vi "Initialize.vi"(8 "error in (no error)":errorcluster, 11 "Software Lock-in in":refnum<class "Software Lock-in.lvclass">) -> (0 "error out":errorcluster, 3 "Software Lock-in out":refnum<class "Software Lock-in.lvclass">)   [LabVIEW 2016, in "Software Lock-in.lvclass"]
uses:
  Software Lock-in.lvclass
  Software Lock-in.lvclass/Software Lock-in.ctl
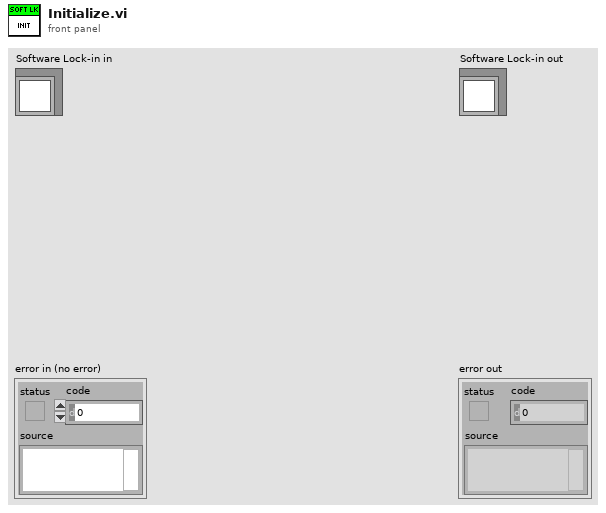
[diagram p1: front panel]
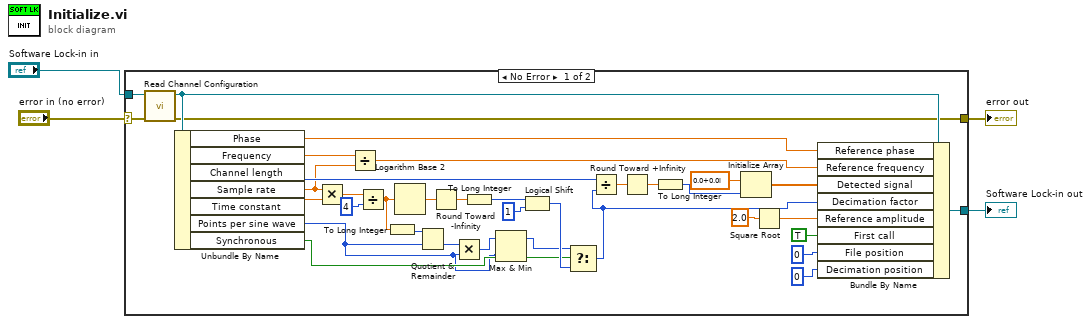
[diagram p0: block diagram]
diagram:
  n1 = case shown="No Error" "error in (no error)" {
    selector: "error in (no error)" -> [w36 w42]
    tunnel: [w25 w42] -> w3
    tunnel: [w39 w41] -> w1
    tunnel: "Software Lock-in in" -> [w40 w41]
    frame No Error {
      n2 = call-dynamic "Read Channel Configuration.vi"("error in (no error)"=w36, "Software Lock-in in"=w40) -> ("error out"=w25:errorcluster, "Software Lock-in out"=w35:refnum<class "Software Lock-in.lvclass">)  [unwired: 8 in]
      n3 = Unbundle By Name(w35) -> ("Phase"=w32:dbl, "Frequency"=w16:dbl, "Channel length"=w24:i64, "Sample rate"=w14:dbl, "Time constant"=w17:dbl, "Points per sine wave"=w7:i32, "Synchronous"=w9:bool)
      n4 = Multiply(x=w14, y=w17) -> (x*y=w31:dbl)
      n5 = Divide(x=w16, y=w14) -> (x/y=w15:dbl)
      n6 = Divide(x=w31, y=4) -> (x/y=w11:dbl)
      n7 = To Long Integer(number=w11) -> (32bit integer=w12:i32)
      n8 = Logarithm Base 2(1:w11) -> (0:w29:dbl)
      n9 = Quotient & Remainder(x=w12, y=w7) -> (floor(x/y)=w10:i32)  [unwired: 1 out]
      n10 = Round Toward -Infinity(1:w29) -> (0:w28:dbl)
      n11 = Multiply(x=w10, y=w7) -> (x*y=w8:i32)
      n12 = To Long Integer(number=w28) -> (32bit integer=w26:i32)
      n13 = Max & Min(x=w8, y=w7) -> (max(x,y)=w6:i32)  [unwired: 1 out]
      n14 = Logical Shift(y=w26, x=1) -> (x << y=w13:i32)
      n15 = Select(t=w6, s=w9, f=w13) -> (s? t:f=w5:i32)
      n16 = Divide(x=w24, y=w5) -> (x/y=w23:dbl)
      n17 = Round Toward +Infinity(x=w23) -> (ceil(x): smallest int >= x=w22:dbl)
      n18 = To Long Integer(number=w22) -> (32bit integer=w19:i32)
      n19 = Initialize Array(cdb 0.0+0.0i ("element"), w19) -> (w20:cdb[])
      n20 = Square Root(x=2.0 ("1/x")) -> (sqrt(x)=w37:dbl)
      n21 = Bundle By Name(cluster=w35, "Reference phase"=w32, "Reference frequency"=w15, "Detected signal"=w20, "Decimation factor"=w5, "Reference amplitude"=w37, "First call"=TRUE, "File position"=i64 0, "Decimation position"=0) -> (w39:refnum<class "Software Lock-in.lvclass">)
    }
    frame Error {
    }
  }
  "error out" <- w3
  "Software Lock-in out" <- w1
